vi "rysowanie.vi"() -> ()   [LabVIEW 2018]
panel:
  in  "Nr":dbl
  in  "Wyjœcie":bool
  in  "Y":dbl(slide) scale=0.0..10.0
  in  "X":dbl(slide) scale=0.0..10.0
  in  "Usuñ ostatni punkt":bool
  in  "Usuñ punkt o numerze":bool
  in  "Rysuj punkt":bool
  out "XY Graph":cluster{"Slide":dbl, "Slide 2":dbl}[](graph)
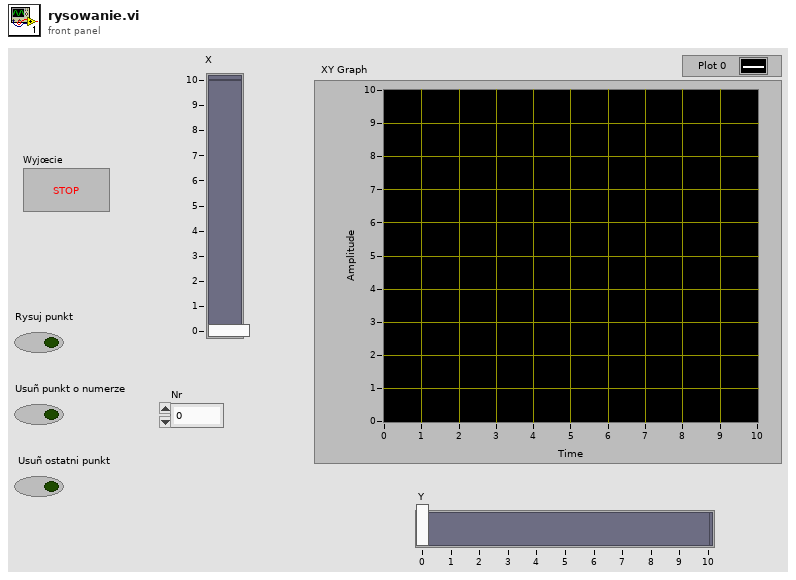
[diagram p1: front panel]
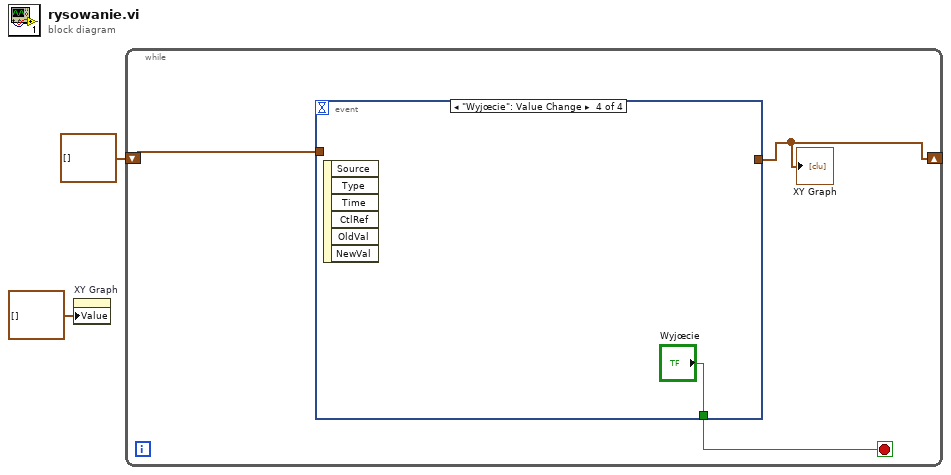
[diagram p0: block diagram]
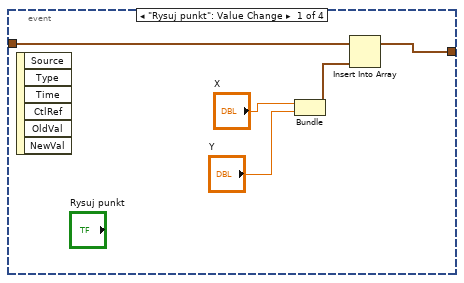
[diagram p2: hidden frame]
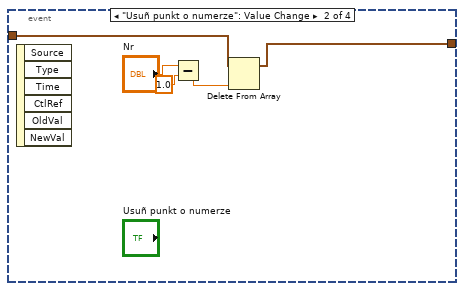
[diagram p3: hidden frame]
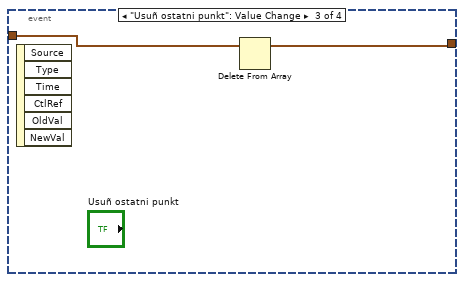
[diagram p4: hidden frame]
diagram:
  n1 = property on="XY Graph" class="XYGraph (strict)"("Value"=cluster{"Slide":dbl, "Slide 2":dbl}[] [] ("XY Graph")) -> ()  [unwired: 2 in, 2 out]
  n2 = while {
    shift-right: [w5] -> _
    shift-left: cluster{"X":dbl, "Y":dbl}[] [] -> [w4]
    stop <- w3 stop-if-true
    n3 = event shown="[3] \"Wyjœcie\": Value Change" {
      selector: _ -> [_ _ _ _]
      dyn-events: _ -> [_ _ _ _]
      timeout: _ -> [_ _ _ _]
      tunnel: [w8 w11 w16 _] -> w5
      tunnel: w4 -> [w6 w15 w17 _]
      tunnel: [_ _ _ "Wyjœcie"] -> w3
      event "Rysuj punkt": Value Change {
        n4 = event-data() -> ()  [unwired: 1 in, 6 out]
        n5 = Bundle("X"="X", "Y"="Y") -> (w7:cluster{"X":dbl, "Y":dbl})  [unwired: 1 in]
        n6 = Insert Into Array(array=w6, new element=w7) -> (w8:cluster{"X":dbl, "Y":dbl}[])  [unwired: 1 in]
      }
      event "Usuñ punkt o numerze": Value Change {
        n7 = event-data() -> ()  [unwired: 1 in, 6 out]
        n8 = Subtract(x="Nr", y=1.0) -> (x-y=w12:dbl)
        n9 = Delete From Array(array=w15, index=w12) -> (array with subset deleted=w11:cluster{"X":dbl, "Y":dbl}[])  [unwired: 1 in, 1 out]
      }
      event "Usuñ ostatni punkt": Value Change {
        n10 = event-data() -> ()  [unwired: 1 in, 6 out]
        n11 = Delete From Array(array=w17) -> (array with subset deleted=w16:cluster{"X":dbl, "Y":dbl}[])  [unwired: 2 in, 1 out]
      }
      event "Wyjœcie": Value Change {
        n12 = event-data() -> ()  [unwired: 1 in, 6 out]
      }
    }
    "XY Graph" <- w5
  }
